vi "Get Histogram.vi"(0 "DeviceIndex":i32) -> (2 "Histogram":u32[](array[numeric]), 3 "IntegralCount":i32, 4 "Overflow":bool)   [LabVIEW 2019]
uses:
  phlib.dll
panel:
  out "Flags":i32 format="%.0b"
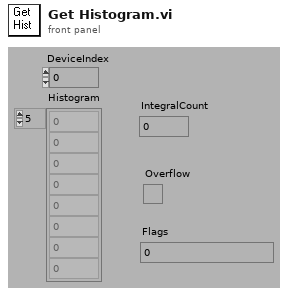
[diagram p1: front panel]
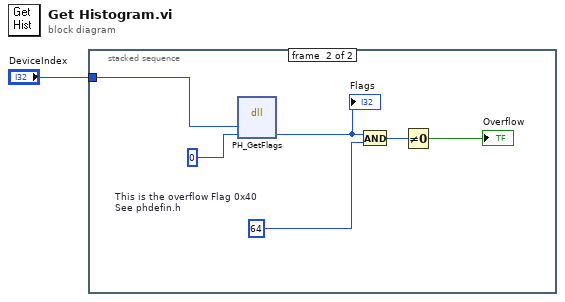
[diagram p0: block diagram]
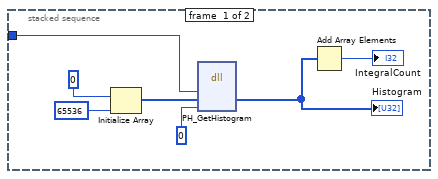
[diagram p2: hidden frame]
diagram:
  n1 = stacked-sequence {
    tunnel: "DeviceIndex" -> [w2 w11]
    frame #0 {
      n2 = Initialize Array "Initialize Array"(u32 0, 65536) -> (w5:u32[])
      n3 = dll-call lib="phlib.dll" fn="PH_GetHistogram"("devidx"=w2, "Chcount"=w5, "block"=u32 0) -> ("Chcount"=w4:u32[])  [unwired: 6 in, 2 out]
      "Histogram" <- w4
      n4 = Add Array Elements(numeric array=w4) -> (sum=→"IntegralCount":u32)
    }
    frame #1 {
      w14 = 64  # This is the overflow Flag 0x40 See phdefin.h
      n5 = dll-call lib="phlib.dll" fn="PH_GetFlags"("devidx"=w11, "flags"=0) -> ("flags"=w9:i32)  [unwired: 5 in, 2 out]
      "Flags" <- w9
      n6 = And(x=w9, y=w14) -> (x .and. y?=w12:i32)
      n7 = Not Equal To 0?(x=w12) -> (x != 0?=→"Overflow":bool)
    }
  }
